vi "ev File path.vi"(8 "error in (no error)":errorcluster, 11 "LF2R IDE in":refnum<class "LF2R IDE.lvclass">) -> (0 "error out":errorcluster, 3 "LF2R IDE out":refnum<class "LF2R IDE.lvclass">)   [LabVIEW 2018, in "LF2R IDE.lvlib" / "LF2R IDE.lvclass"]
uses:
  LF2R IDE.lvclass
  LF2R IDE.lvclass/LF2R IDE.ctl
  ScintillaNET/ScintillaNET.lvclass
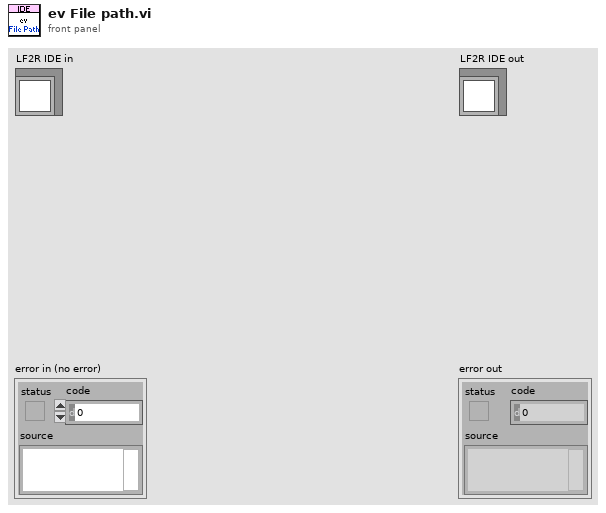
[diagram p1: front panel]
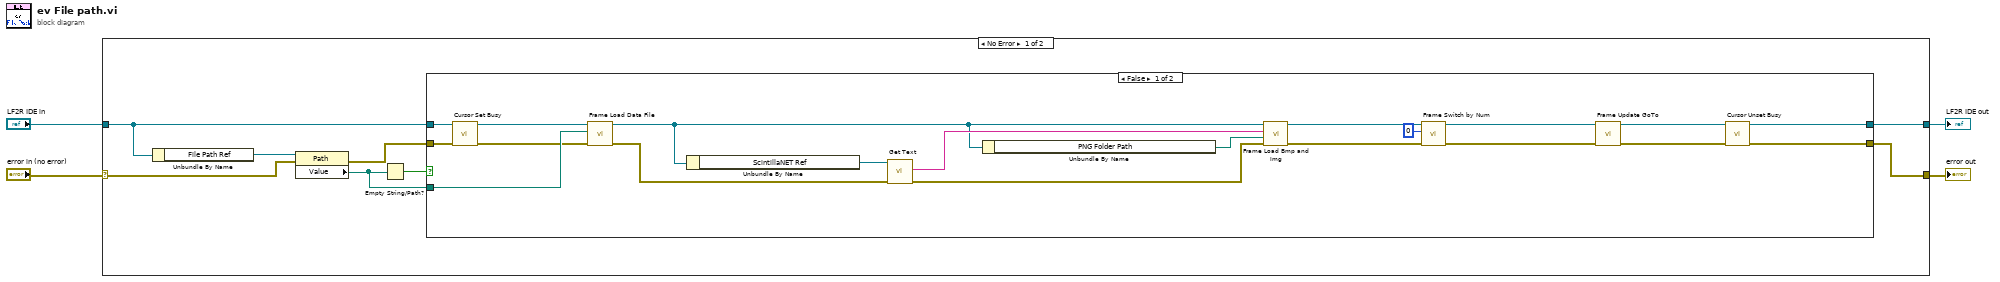
[diagram p0: block diagram]
diagram:
  n1 = case shown="No Error" "error in (no error)" {
    selector: "error in (no error)" -> [w8 w36]
    tunnel: [w11 w36] -> w3
    tunnel: [w12 w35] -> w1
    tunnel: "LF2R IDE in" -> [w10 w35]
    frame No Error {
      n2 = Unbundle By Name(w10) -> ("File Path Ref"=w9:refnum<vi>)
      n3 = property class="Path"(reference=w9, error in=w8) -> (error out=w5:errorcluster, "Value"=w6:path)  [unwired: 1 out]
      n4 = Empty String/Path?(string/path=w6) -> (empty?=w7:bool)
      n5 = case shown="False" w7 {
        tunnel: [w21 w34] -> w12
        tunnel: [w22 w33] -> w11
        tunnel: w10 -> [w25 w34]
        tunnel: w5 -> [w26 w33]
        tunnel: w6 -> [w32 _]
        frame False {
          n6 = call "Cursor Set Busy.vi"("error in (no error)"=w26, "LF2R IDE in"=w25) -> ("error out"=w27:errorcluster, "LF2R IDE out"=w28:refnum<class "LF2R IDE.lvclass">)  [unwired: 8 in]
          n7 = call "Frame Load Data File.vi"("error in (no error)"=w27, "File Path"=w32, "IDE simple in"=w28) -> ("error out"=w30:errorcluster, "IDE simple out"=w14:refnum<class "LF2R IDE.lvclass">)  [unwired: 7 in]
          n8 = Unbundle By Name(w14) -> ("ScintillaNET Ref"=w31:refnum<class "ScintillaNET.lvclass">)
          n9 = call "Get Text.vi"("error in (no error)"=w30, "ScintillaNET in"=w31) -> ("error out"=w15:errorcluster, "Text"=w29:string)  [unwired: 7 in, 1 out]
          n10 = Unbundle By Name(w14) -> ("PNG Folder Path"=w13:path)
          n11 = call "Frame Load Bmp and Img.vi"("error in (no error)"=w15, "PNG Path"=w13, "File String"=w29, "LF2R IDE in"=w14) -> ("error out"=w19:errorcluster, "LF2R IDE out"=w20:refnum<class "LF2R IDE.lvclass">)  [unwired: 6 in]
          n12 = call "Frame Switch by Num.vi"("error in (no error)"=w19, "Frame Num"=u32 0, "LF2R IDE in"=w20) -> ("error out"=w17:errorcluster, "LF2R IDE out"=w18:refnum<class "LF2R IDE.lvclass">)  [unwired: 7 in]
          n13 = call "Frame Update GoTo.vi"("error in (no error)"=w17, "LF2R IDE in"=w18) -> ("error out"=w23:errorcluster, "LF2R IDE out"=w24:refnum<class "LF2R IDE.lvclass">)  [unwired: 8 in]
          n14 = call "Cursor Unset Busy.vi"("error in (no error)"=w23, "LF2R IDE in"=w24) -> ("error out"=w22:errorcluster, "LF2R IDE out"=w21:refnum<class "LF2R IDE.lvclass">)  [unwired: 8 in]
        }
        frame True {
        }
      }
    }
    frame Error {
    }
  }
  "error out" <- w3
  "LF2R IDE out" <- w1
